vi "Get Module Connection Information.vi"(8 "error in (no error)":errorcluster, 11 "Routing and Faulting Custom Device Ref in":T3 format="%.0x") -> (0 "error out":errorcluster, 2 "Module Connection Information":T1[](array[typedef]), 3 "Routing and Faulting Custom Device Ref out":T3 format="%.0x")   [LabVIEW 2017, in "Routing and Faulting Scripting.lvlib"]
uses:
  Routing and Faulting Scripting.lvlib
  <vilib>/NI Veristand/Custom Device API/Custom Device Item Ref.ctl
  Types/Module Connection Information.ctl
  Shared/Routing and Faulting Hardware API/Types/Possible Connections for Endpoint.ctl
  Shared/Routing and Faulting Hardware API/Routing and Faulting Hardware API.lvlib
  <vilib>/NI Veristand/Custom Device API/Custom Device API.lvlib
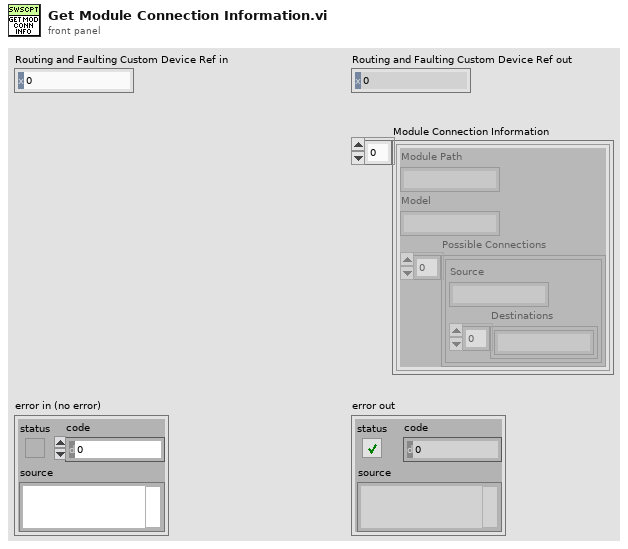
[diagram p1: front panel]
types:
  T1 = typedef "Routing and Faulting Scripting.lvlib/Module Connection Information.ctl" = cluster{"Module Path":string, "Model":string, "Possible Connections":T2[]}
  T2 = typedef "Routing and Faulting Hardware API.lvlib/Possible Connections for Endpoint.ctl" = cluster{"Source":string, "Destinations":string[]}
  T3 = typedef "Custom Device API.lvlib/Custom Device Item Ref.ctl" = u64
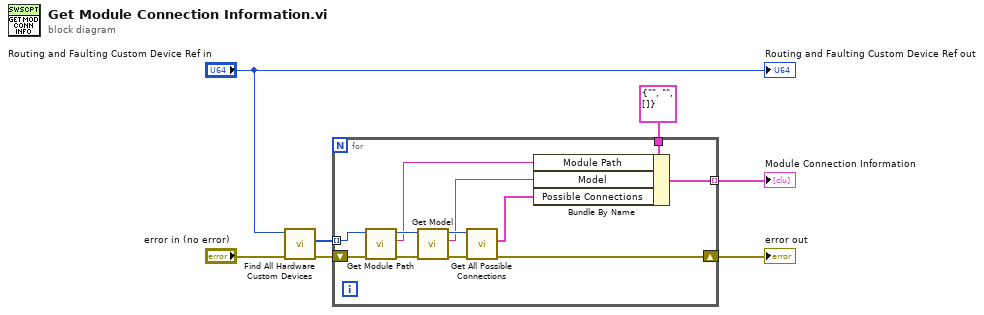
[diagram p0: block diagram]
diagram:
  n1 = call "Find All Hardware Custom Devices.vi"("error in (no error)"="error in (no error)", "Routing and Faulting Ref in"="Routing and Faulting Custom Device Ref in") -> ("error out"=w6:errorcluster, "Hardware Refs"=w5:T3[])  [unwired: 7 in, 1 out]
  n2 = for {
    shift-right: [w16] -> w1
    shift-left: w6 -> [w19]
    tunnel: w5 -> [w15] mode=indexing
    tunnel: T1 {"Module Path"="", "Model"="", "Possible Connections"=[]} ("Module Connection Information") -> [w14]
    tunnel: [w8] -> w2 mode=indexing
    n3 = call "Get Module Path.vi"("error in (no error)"=w19, "Hardware Ref in"=w15) -> ("error out"=w18:errorcluster, "Module Path"=w11:string, "Hardware Ref out"=w13:T3)  [unwired: 6 in, 1 out]
    n4 = call "Get Model.vi"("error in (no error)"=w18, "Hardware Ref in"=w13) -> ("error out"=w17:errorcluster, "Model"=w10:string, "Hardware Ref out"=w12:T3)  [unwired: 6 in, 1 out]
    n5 = call "Get All Possible Connections.vi"("error in (no error)"=w17, "Hardware Ref in"=w12) -> ("error out"=w16:errorcluster, "Possible Connections"=w9:T2[])  [unwired: 6 in, 2 out]
    n6 = Bundle By Name(cluster=w14, "Module Path"=w11, "Model"=w10, "Possible Connections"=w9) -> (w8:T1)
  }
  "Module Connection Information" <- w2
  "error out" <- w1
  "Routing and Faulting Custom Device Ref out" <- "Routing and Faulting Custom Device Ref in"
